vi "FTW-Reflection-Type.vi"(7 "Anything":variant) -> (6 "Data Name":string, 8 "LabVIEW Type":T1, 10 "Inner Type for composite Data Types":variant)   [LabVIEW 2012]
uses:
  FTW-Reflection-Types.ctl
panel:
  # "Inputs"
  # "Outputs"
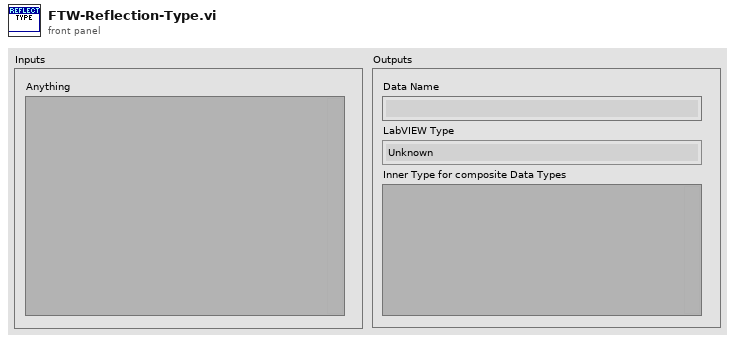
[diagram p1: front panel]
types:
  T1 = typedef "FTW-Reflection-Types.ctl" = enum16{"Unknown", "Void", "Array", "Cluster", "LVObject", "Boolean", "I8", "I16", "I32", "I64", "U8", "U16", "U32", "U64", "SGL", "DBL", "EXT", "CSG", "CDB", "CXT", "FXP", "EnumU8", "EnumU16", "EnumU32", "EnumU64", "SGLwithUnit", "DBLwithUnit", "EXTwithUnit", "CSGwithUnit", "CDBwithUnit", "CXTwithUnit", "String", "Path", "Picture", "Tag", "LVVariant", "Timestamp", "WaveformI8", "WaveformI16", "WaveformI32", "WaveformI64", "WaveformU8", "WaveformU16", "WaveformU32", "WaveformU64", "WaveformSGL", "WaveformDBL", "WaveformEXT", "WaveformCSG", "WaveformCDB", "WaveformCXT", "WaveformDigital", "WaveformUnknownType", "DigitalData", "DynamicData", "ExternalData", "FileByteStream", "TDMStream", "dotNET", "ActiveX", "VIServerReference", "VIReference", "ApplicationInstance", "Menu", "ConnectionDataSocket", "ConnectionVISA", "ConnectionBluetooth", "ConnectionIrDA", "ConnectionTCP", "ConnectionUDP", "ConnectionHTTPClient", "ConnectionFTP", "Occurrence", "Notifier", "Queue", "Rendezvous", "Semaphore", "RTFIFO", "EventPublisher", "EventRegistration", "EventCallback", "DataValueReference", "GenericClass", "GenericClassTag", "GenericClassDeepCopy", "GenericClassFlattened", "GenericClassTagFlattened", "GenericReferenceType", "WindowsRegistry", "OverloadedDatalogRef", "ReferenceUnknownType"}
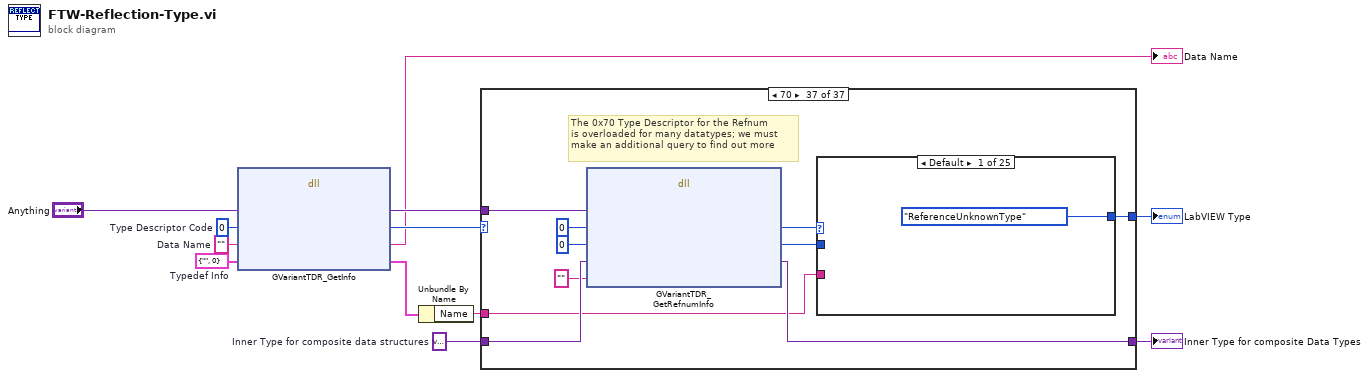
[diagram p0: block diagram]
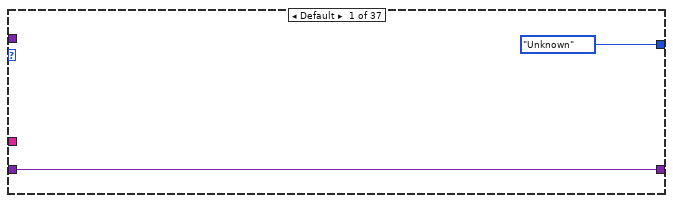
[diagram p2: hidden frame]
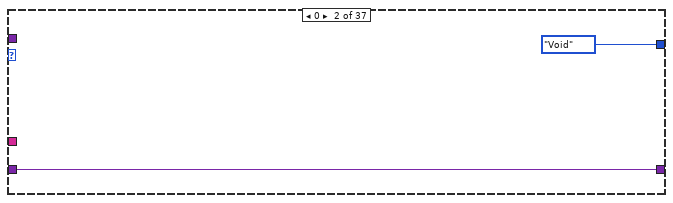
[diagram p3: hidden frame]
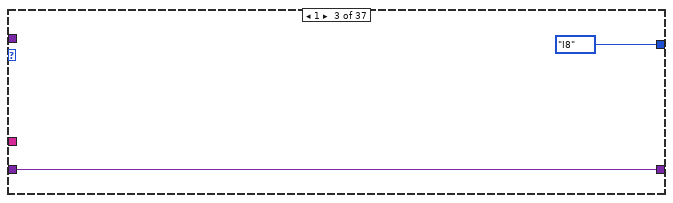
[diagram p4: hidden frame]
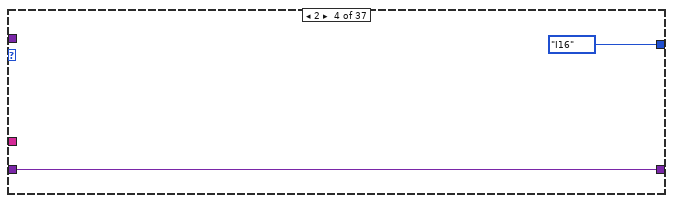
[diagram p5: hidden frame]
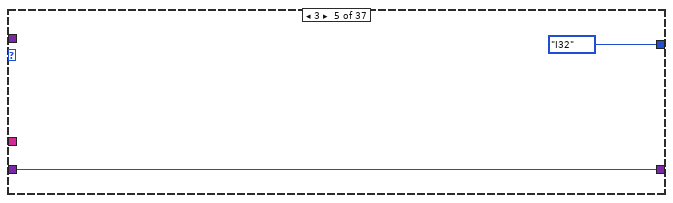
[diagram p6: hidden frame]
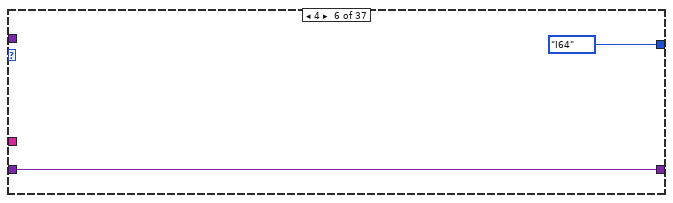
[diagram p7: hidden frame]
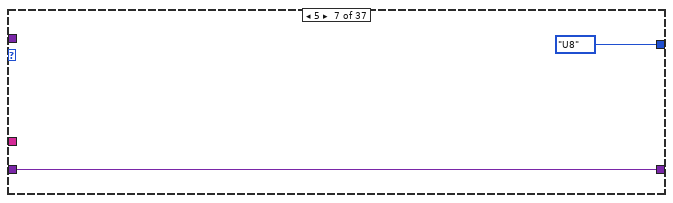
[diagram p8: hidden frame]
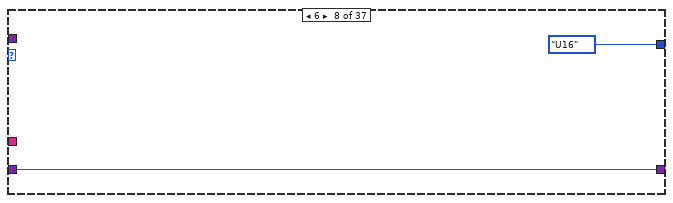
[diagram p9: hidden frame]
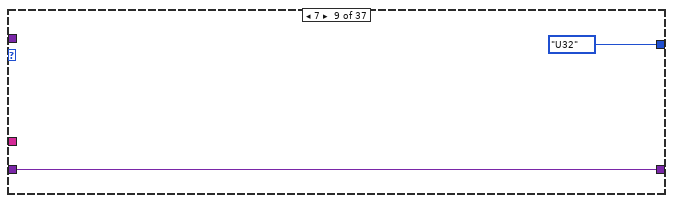
[diagram p10: hidden frame]
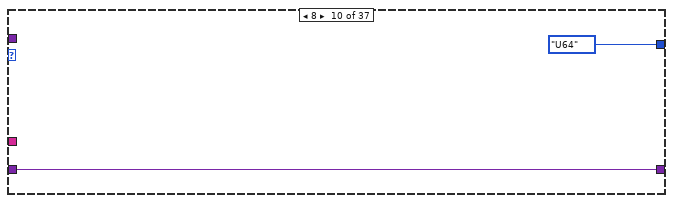
[diagram p11: hidden frame]
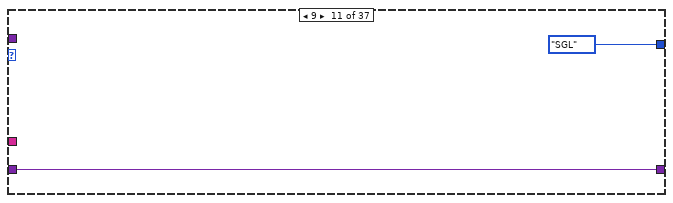
[diagram p12: hidden frame]
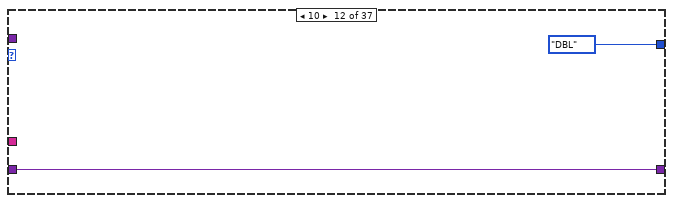
[diagram p13: hidden frame]
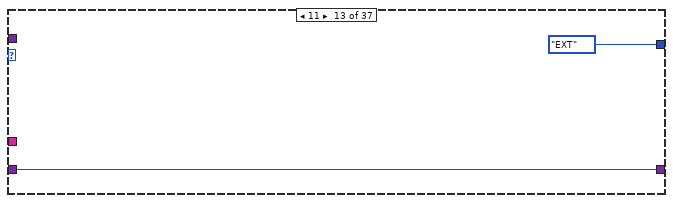
[diagram p14: hidden frame]
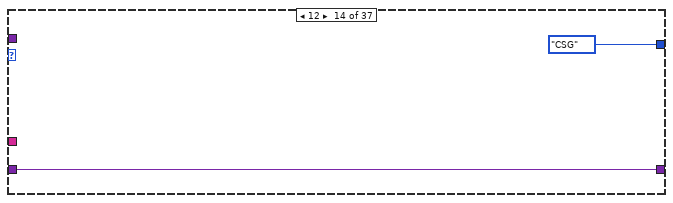
[diagram p15: hidden frame]
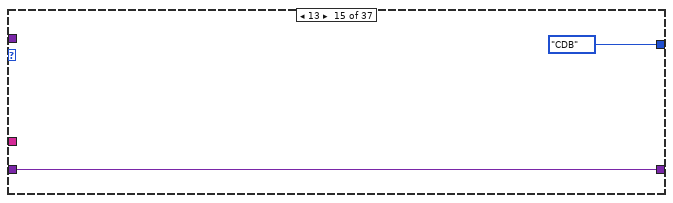
[diagram p16: hidden frame]
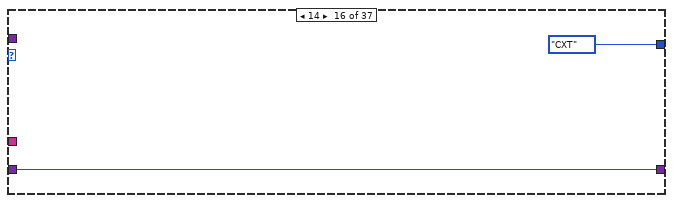
[diagram p17: hidden frame]
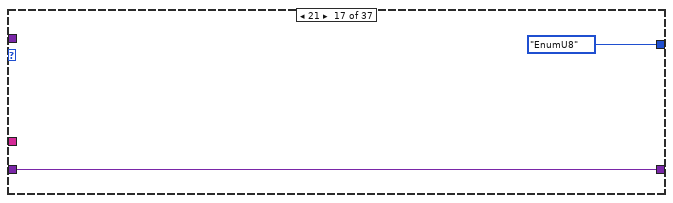
[diagram p18: hidden frame]
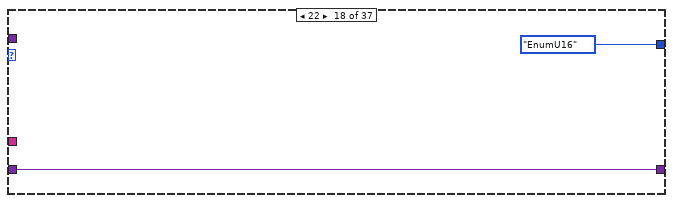
[diagram p19: hidden frame]
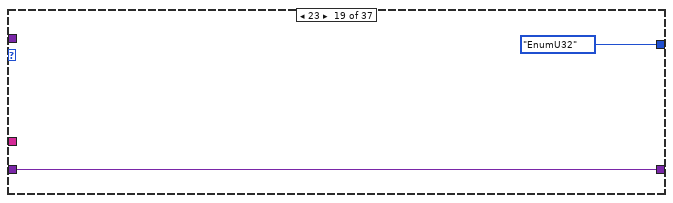
[diagram p20: hidden frame]
diagram:
  w4 = variant  # Inner Type for composite data structures
  w9 = i16 0  # Type Descriptor Code
  w10 = cluster{"Name":string, "Timestamp":u32} {"Name"="", "Timestamp"=0}  # Typedef Info
  w11 = ""  # Data Name
  n1 = dll-call lib="LabVIEW" fn="GVariantTDR_GetInfo"("Variant"="Anything", "Type Descriptor Code"=w9, "Data Name"=w11, "Typedef Info"=w10) -> ("Variant"=w5:variant, "Type Descriptor Code"=w8:i16, "Data Name"=→"Data Name":string, "Typedef Info"=w6:cluster{"Name":string, "Timestamp":u32})  [unwired: 3 in, 3 out]
  n2 = Unbundle By Name(w6) -> ("Name"=w2:string)
  n3 = case shown="70" w8 {
    tunnel: [FTW-Reflection-Types."Unknown" FTW-Reflection-Types."Void" FTW-Reflection-Types."I8" FTW-Reflection-Types."I16" FTW-Reflection-Types."I32" FTW-Reflection-Types."I64" FTW-Reflection-Types."U8" FTW-Reflection-Types."U16" FTW-Reflection-Types."U32" FTW-Reflection-Types."U64" FTW-Reflection-Types."SGL" FTW-Reflection-Types."DBL" FTW-Reflection-Types."EXT" FTW-Reflection-Types."CSG" FTW-Reflection-Types."CDB" FTW-Reflection-Types."CXT" FTW-Reflection-Types."EnumU8" FTW-Reflection-Types."EnumU16" FTW-Reflection-Types."EnumU32" FTW-Reflection-Types."EnumU64" FTW-Reflection-Types."SGLwithUnit" FTW-Reflection-Types."DBLwithUnit" FTW-Reflection-Types."EXTwithUnit" FTW-Reflection-Types."CSGwithUnit" FTW-Reflection-Types."CDBwithUnit" FTW-Reflection-Types."CXTwithUnit" FTW-Reflection-Types."Boolean" FTW-Reflection-Types."String" FTW-Reflection-Types."Path" FTW-Reflection-Types."Picture" FTW-Reflection-Types."Tag" FTW-Reflection-Types."Cluster" FTW-Reflection-Types."LVVariant" FTW-Reflection-Types."FXP" FTW-Reflection-Types."Array" w88 w120] -> w7
    tunnel: w5 -> [_ _ _ _ _ _ _ _ _ _ _ _ _ _ _ _ _ _ _ _ _ _ _ _ _ _ _ _ _ _ _ _ _ _ w84 w91 w119]
    tunnel: w4 -> [w13 w15 w17 w19 w21 w23 w25 w27 w29 w31 w33 w35 w37 w39 w41 w43 w45 w47 w49 w51 w53 w55 w57 w59 w61 w63 w65 w67 w69 w71 w73 w75 w77 w79 w83 w87 w117]
    tunnel: [w13 w15 w17 w19 w21 w23 w25 w27 w29 w31 w33 w35 w37 w39 w41 w43 w45 w47 w49 w51 w53 w55 w57 w59 w61 w63 w65 w67 w69 w71 w73 w75 w77 w79 w82 w86 w116] -> w3
    tunnel: w2 -> [_ _ _ _ _ _ _ _ _ _ _ _ _ _ _ _ _ _ _ _ _ _ _ _ _ _ _ _ _ _ _ _ _ _ _ _ w113]
    frame Default {
    }
    frame 0 {
    }
    frame 1 {
    }
    frame 2 {
    }
    frame 3 {
    }
    frame 4 {
    }
    frame 5 {
    }
    frame 6 {
    }
    frame 7 {
    }
    frame 8 {
    }
    frame 9 {
    }
    frame 10 {
    }
    frame 11 {
    }
    frame 12 {
    }
    frame 13 {
    }
    frame 14 {
    }
    frame 21 {
    }
    frame 22 {
    }
    frame 23 {
    }
    frame 24 {
    }
    frame 25 {
    }
    frame 26 {
    }
    frame 27 {
    }
    frame 28 {
    }
    frame 29 {
    }
    frame 30 {
    }
    frame 33 {
    }
    frame 48 {
    }
    frame 50 {
    }
    frame 51 {
    }
    frame 55 {
    }
    frame 80 {
    }
    frame 83 {
    }
    frame 95 {
    }
    frame 64 {
      # "Let's query the 0x40 Type Descriptor\n(Array Type) for it's element data type."
      n4 = dll-call lib="LabVIEW" fn="GVariantTDR_GetArrayInfo"("Variant"=w84, "Element Type"=w83, "Dimensions"=i32[] []) -> ("Element Type"=w82:variant)  [unwired: 6 in, 2 out]
    }
    frame 84 {
      # "The 0x54 Type Descriptor for the Waveform\nis overloaded for many datatypes; we must\nmake an additional query to find out more"
      n5 = dll-call lib="LabVIEW" fn="GVariantTDR_GetMDTInfo"("Variant"=w91, "Waveform Type"=i16 0, "Inner Type"=w87) -> ("Waveform Type"=w89:i16, "Inner Type"=w86:variant)  [unwired: 4 in, 3 out]
      n6 = case shown="Default" w89 {
        tunnel: [FTW-Reflection-Types."WaveformUnknownType" FTW-Reflection-Types."WaveformI16" FTW-Reflection-Types."WaveformDBL" FTW-Reflection-Types."WaveformSGL" FTW-Reflection-Types."Timestamp" FTW-Reflection-Types."DigitalData" FTW-Reflection-Types."WaveformDigital" FTW-Reflection-Types."DynamicData" FTW-Reflection-Types."WaveformEXT" FTW-Reflection-Types."WaveformU8" FTW-Reflection-Types."WaveformU16" FTW-Reflection-Types."WaveformU32" FTW-Reflection-Types."WaveformI8" FTW-Reflection-Types."WaveformI32" FTW-Reflection-Types."WaveformCSG" FTW-Reflection-Types."WaveformCDB" FTW-Reflection-Types."WaveformCXT" FTW-Reflection-Types."WaveformI64" FTW-Reflection-Types."WaveformU64"] -> w88
        frame Default {
        }
        frame 2 {
        }
        frame 3 {
        }
        frame 5 {
        }
        frame 6 {
        }
        frame 7 {
        }
        frame 8 {
        }
        frame 9 {
        }
        frame 10 {
        }
        frame 11 {
        }
        frame 12 {
        }
        frame 13 {
        }
        frame 14 {
        }
        frame 15 {
        }
        frame 16 {
        }
        frame 17 {
        }
        frame 18 {
        }
        frame 19 {
        }
        frame 20 {
        }
      }
    }
    frame 112 {
      # "The 0x70 Type Descriptor for the Refnum\nis overloaded for many datatypes; we must\nmake an additional query to find out more"
      n7 = dll-call lib="LabVIEW" fn="GVariantTDR_GetRefnumInfo"("Variant"=w119, "Refnum Kind"=i16 0, "Refnum Subkind"=0, "Inner Type"=w117, "Information"="") -> ("Refnum Kind"=w118:i16, "Refnum Subkind"=w111:i32, "Inner Type"=w116:variant)  [unwired: 4 in, 4 out]
      n8 = case shown="Default" w118 {
        tunnel: [FTW-Reflection-Types."ReferenceUnknownType" FTW-Reflection-Types."GenericReferenceType" w124 FTW-Reflection-Types."FileByteStream" FTW-Reflection-Types."Occurrence" w133 FTW-Reflection-Types."ActiveX" w138 FTW-Reflection-Types."Menu" FTW-Reflection-Types."ConnectionDataSocket" FTW-Reflection-Types."ConnectionVISA" FTW-Reflection-Types."ConnectionUDP" FTW-Reflection-Types."Notifier" FTW-Reflection-Types."Queue" FTW-Reflection-Types."ConnectionIrDA" FTW-Reflection-Types."GenericClass" FTW-Reflection-Types."GenericClassTag" FTW-Reflection-Types."EventRegistration" FTW-Reflection-Types."dotNET" FTW-Reflection-Types."EventPublisher" FTW-Reflection-Types."EventCallback" FTW-Reflection-Types."LVObject" FTW-Reflection-Types."ConnectionBluetooth" FTW-Reflection-Types."DataValueReference" FTW-Reflection-Types."TDMStream"] -> w120
        tunnel: w113 -> [_ _ w123 _ _ w132 _ _ _ _ _ _ _ _ _ _ _ _ _ _ _ _ _ _ _]
        tunnel: w111 -> [_ _ _ _ _ _ _ w137 _ _ _ _ _ _ _ _ _ _ _ _ _ _ _ _ _]
        frame Default {
        }
        frame 0 {
        }
        frame 1 {
          n9 = case shown="Default" w123 {
            tunnel: [FTW-Reflection-Types."OverloadedDatalogRef" FTW-Reflection-Types."Semaphore" FTW-Reflection-Types."Rendezvous" FTW-Reflection-Types."WindowsRegistry" FTW-Reflection-Types."ConnectionHTTPClient"] -> w124
            frame Default {
            }
            frame "Semaphore RefNum" {
            }
            frame "Rendezvous RefNum" {
            }
            frame "Registry refnum.ctl" {
            }
            frame "LabVIEWHTTPClient.lvlib:ClientHandle.ctl" {
            }
          }
        }
        frame 2 {
        }
        frame 4 {
        }
        frame 5 {
          n10 = case shown="Default" w132 {
            tunnel: [FTW-Reflection-Types."ConnectionTCP" FTW-Reflection-Types."ConnectionFTP"] -> w133
            frame Default {
            }
            frame "NI_FTP.lvlib:FTP Session.ctl" {
            }
          }
        }
        frame 7 {
        }
        frame 8 {
          n11 = case shown="Default" w137 {
            tunnel: [FTW-Reflection-Types."VIServerReference" FTW-Reflection-Types."ApplicationInstance" FTW-Reflection-Types."VIReference"] -> w138
            frame Default {
            }
            frame 1 {
            }
            frame 2 {
            }
          }
        }
        frame 9 {
        }
        frame 13 {
        }
        frame 14 {
        }
        frame 16 {
        }
        frame 17 {
        }
        frame 18 {
        }
        frame 19 {
        }
        frame 20 {
        }
        frame 21 {
        }
        frame 23 {
        }
        frame 24 {
        }
        frame 25 {
        }
        frame 27 {
        }
        frame 30 {
        }
        frame 31 {
        }
        frame 32 {
        }
        frame 34 {
        }
      }
    }
  }
  "LabVIEW Type" <- w7
  "Inner Type for composite Data Types" <- w3
